vi "NI6602.Reset Channel Values.vi"(0 "i ref in":refnum<vi>, 5 "error in (no error)":errorcluster) -> (14 "i ref out":refnum<vi>, 19 "error out":errorcluster)   [LabVIEW 2014, in "NI6602.lvlib"]
doc: "Resets the internal counters to 0.\n\nLicense Agreement for this software:\n\nCopyright (C)\nGesellschaft für Schwerionenforschung, GSI\nPlanckstr. 1\n64291 Darmstadt\nGermany\n\nContact: D.Beck@gsi.de \n\nThis program is free software; you can redistribute it and/or modify it under the terms of the \nGNU General Public License as published by the Free Software Foundation; either version 2 of \nthe license, or (at your option) any later version.\n\nThis program is distributed in the hope that it will be useful, but WITHOUT ANY WARRANTY; \nwithout even the implied warranty of MERCHANTABILITY or FITNESS FOR A PARTICULAR PURPOSE. See the GNU General License for more details (http://www.gnu.org).\n\nGesellschaft für Schwerionenforschung, GSI\nPlanckstr. 1, 64291 Darmstadt, Germany\nFor all questions and ideas contact: M.Richter@gsi.de, H.Brand@gsi.de or D.Beck@gsi.de.\nLast update: 16-JUN-2004"
uses:
  NI6602.lvlib
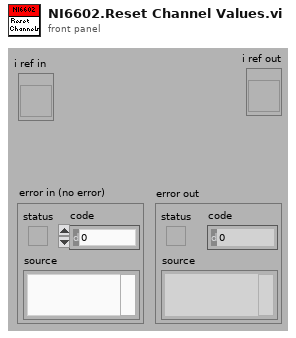
[diagram p1: front panel]
types:
  T1 = typedef "NI6602.lvlib/NI6602.i attribute.ctl" = cluster{"CounterDAQ Channels":cluster{"task":refnum<k21>, "Channel Name":string}[], "RateServiceIDs":i32[], "Running?":bool, "IntegralServiceIDs":i32[], "ThresholdID":i32, "Threshold":dbl, "IntegralValues":dbl[], "Stopped?":bool}
  T2 = cluster{"task":refnum<k21>, "Channel Name":string}[]
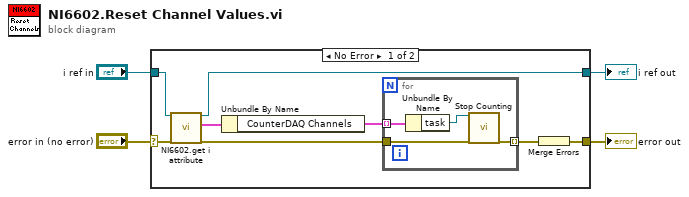
[diagram p0: block diagram]
diagram:
  n1 = case shown="No Error" "error in (no error)" {
    selector: "error in (no error)" -> [w11 w18]
    tunnel: [w6 w17] -> w4
    tunnel: [w5 w18] -> w3
    tunnel: "i ref in" -> [w9 w17]
    frame No Error {
      n2 = call "NI6602.get i attribute.vi"("i ref in"=w9, "error in (no error)"=w11) -> ("i ref out"=w6:refnum<vi>, "i attribute"=w8:T1, "error out"=w10:errorcluster)  [unwired: 15 in]
      n3 = Unbundle By Name(w8) -> ("CounterDAQ Channels"=w7:T2)
      n4 = for {
        tunnel: w10 -> [w16]
        tunnel: [w15] -> w12 mode=indexing
        tunnel: w7 -> [w14] mode=indexing
        n5 = Unbundle By Name(w14) -> ("task"=w13:refnum<k21>)
        n6 = call "Stop Counting.vi"("task/channels in"=w13, "error in"=w16) -> ("error out"=w15:errorcluster)  [unwired: 16 in, 1 out]
      }
      n7 = Merge Errors(w12) -> (w5:errorcluster)
    }
    frame Error {
    }
  }
  "i ref out" <- w4
  "error out" <- w3
